vi "LDLT-Decomposition.vi"(11 "Input Matrix":T1) -> (2 "D":T1, 3 "L":T1)   [LabVIEW 2019]
doc: "This VI computes the square root free Cholesky factorization\n\n A=L*D*L'\n\nWhere L is a lower triangular matrix with ones on the diagonal, and D is a diagonal matrix. \nIt is assumed that A is symmetric and postive definite.\nReference: Golub and Van Loan, \"Matrix Computations\", second edition, p 137. \nit is based in the work made by Brian Borchers (borchers@nmt.edu) in MATLAB.\n\nCreated by Davis Montenegro\n10-05-2013"
uses:
  <vilib>/Analysis/Matrix/Datatypes/RealMatrix.ctl
  <vilib>/Analysis/Matrix/Numeric/Conversions/Matrix To Array - RM.vi
  <vilib>/Analysis/Matrix/Numeric/Conversions/Array To Matrix - RA.vi
  <vilib>/Analysis/Matrix/Numeric/Multiply/Multiply - RM,RM.vi
  <vilib>/Analysis/Matrix/Numeric/Subtract/Subtract (Elementwise) - R,RM.vi
  <vilib>/Analysis/Matrix/Numeric/Conversions/Array To Matrix - RA2.vi
  <vilib>/Analysis/Matrix/Numeric/Subtract/Subtract - RM,RM.vi
  <vilib>/Analysis/Matrix/NI_Matrix.lvlib
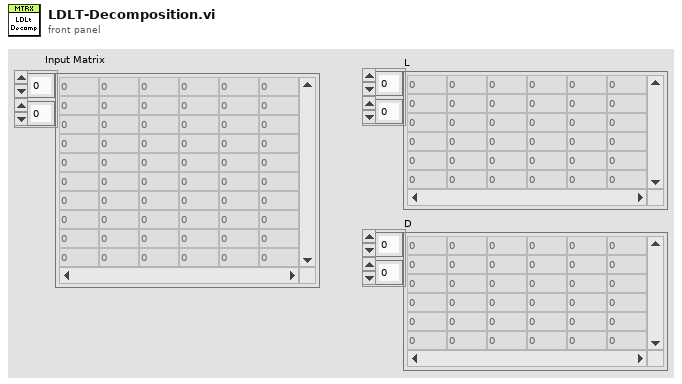
[diagram p1: front panel]
types:
  T1 = typedef "NI_Matrix.lvlib/RealMatrix.ctl" = dbl[][]
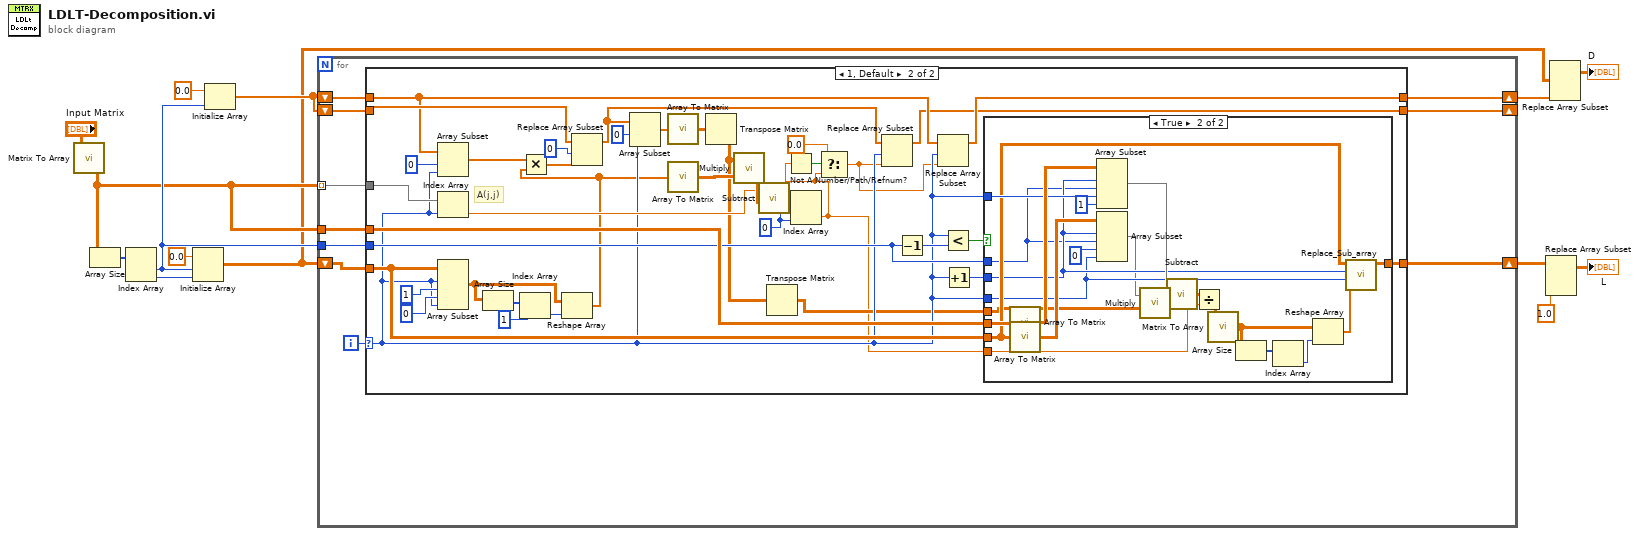
[diagram p0: block diagram]
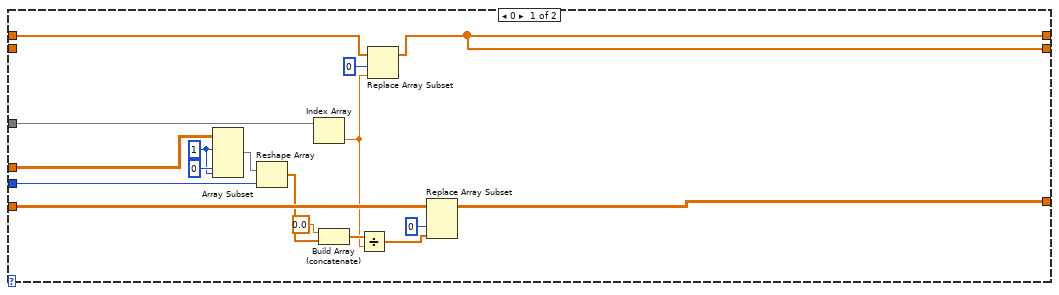
[diagram p2: hidden frame]
diagram:
  n1 = call-poly <vilib>:"Matrix To Array.vi"("Real Matrix"="Input Matrix") -> ("Real 2D Array"=w5:dbl[][])
  n2 = Array Size(array=w5) -> (size(s)=w14:i32[])
  n3 = Index Array(array=w14) -> (element #1=w10:i32, element #2=w13:i32)  [unwired: 2 in]
  n4 = Initialize Array(0.0, w10, w13) -> (w2:dbl[][])
  n5 = Initialize Array(0.0, w10) -> (w7:dbl[])
  n6 = for {
    tunnel: w5 -> [w23] mode=indexing
    shift-right: [w16] -> _
    shift-left: w7 -> [w22]
    shift-right: [w15] -> w3
    shift-left: w7 -> [w21]
    tunnel: w5 -> [w19]
    tunnel: w10 -> [w18]
    shift-right: [w17] -> w9
    shift-left: w2 -> [w20]
    i -> [w24]
    n7 = case shown="1, Default" w24 {
      selector: w24 -> [_ w52]
      tunnel: w23 -> [w41 w76]
      tunnel: w22 -> [_ w75]
      tunnel: w21 -> [w28 w68]
      tunnel: [w25 w67] -> w15
      tunnel: [w25 w50] -> w16
      tunnel: w20 -> [w37 w58]
      tunnel: w19 -> [w40 w65]
      tunnel: w18 -> [w33 w53]
      tunnel: [w31 w62] -> w17
      frame 0 {
        w38 = 1 ("index")
        n8 = Array Subset(array=w40, index (row)=w38, index (col)=0 ("index"), length (col)=w38) -> (w34:dbl[][])  [unwired: 1 in]
        n9 = Reshape Array(w34, w33) -> (w32:dbl[])
        n10 = Index Array(array=w41) -> (element=w26:dbl)  [unwired: 1 in]
        n11 = Build Array (concatenate)(0.0, w32) -> (w30:dbl[])
        n12 = Divide(x=w30, y=w26) -> (x/y=w29:dbl[])
        n13 = Replace Array Subset(array=w28, new element=w26, index=0 ("index (row)")) -> (w25:dbl[])
        n14 = Replace Array Subset(array=w37, new element=w29, index (col)=0 ("disabled index (col)")) -> (w31:dbl[][])  [unwired: 1 in]
      }
      frame 1, Default {
        w69 = 0 ("index (row)")
        # "A(j,j)"
        n15 = Array Subset(array=w68, index=0, length=w52) -> (w80:dbl[])
        n16 = Index Array(array=w76, index=w52) -> (element=w71:dbl)
        n17 = Array Subset(array=w58, index (row)=w52, length (row)=1 ("length"), index (col)=0 ("length"), length (col)=w52) -> (w77:dbl[][])
        n18 = Array Size(array=w77) -> (size(s)=w79:i32[])
        n19 = Index Array(array=w79, index=1) -> (element=w78:i32)
        n20 = Reshape Array(w77, w78) -> (w42:dbl[])
        n21 = Multiply(x=w80, y=w42) -> (x*y=w74:dbl[])
        n22 = Replace Array Subset(array=w75, new element=w74, index=0) -> (w56:dbl[])
        n23 = Array Subset(array=w56, index=0, length=w52) -> (w54:dbl[])
        n24 = call-poly <vilib>:"Array To Matrix.vi"("Real 1D Array"=w54) -> ("Real Matrix (Column Vector)"=w57:T1)
        n25 = call-poly <vilib>:"Array To Matrix.vi"("Real 1D Array"=w42) -> ("Real Matrix (Column Vector)"=w49:T1)
        n26 = Transpose Matrix(1:w57) -> (0:w48:T1)
        n27 = call-poly <vilib>:"Multiply.vi"("Real Matrix B"=w49, "Real Matrix A"=w48) -> ("A * B"=w72:T1)
        n28 = call-poly <vilib>:"Subtract.vi"("Real Matrix A"=w72, "Real Scalar c"=w71) -> ("c - A"=w70:T1)
        n29 = Transpose Matrix(1:w48) -> (0:w47:T1)
        n30 = Index Array(array=w70, index (row)=w69, index (col)=w69) -> (element=w44:dbl)
        n31 = Not A Number/Path/Refnum?(number/path/refnum=w44) -> (NaN/Path/Refnum?=w45:bool)
        n32 = Select(t=0.0, s=w45, f=w44) -> (s? t:f=w43:dbl)
        n33 = Replace Array Subset(array=w56, new element=w43, index=w52) -> (w50:dbl[])
        n34 = Decrement(x=w53) -> (x-1=w63:i32)
        n35 = Replace Array Subset(array=w68, new element=w43, index=w52) -> (w67:dbl[])
        n36 = Less?(x=w52, y=w63) -> (x < y?=w66:bool)
        n37 = Increment(x=w52) -> (x+1=w64:i32)
        n38 = case shown="True" w66 {
          tunnel: w58 -> [w81 w87]
          tunnel: w65 -> [_ w101]
          tunnel: w47 -> [_ w83]
          tunnel: w52 -> [_ w85]
          tunnel: w64 -> [_ w86]
          tunnel: w52 -> [_ w99]
          tunnel: w44 -> [_ w97]
          tunnel: [w81 w89] -> w62
          tunnel: w53 -> [_ w82]
          frame False {
          }
          frame True {
            n39 = call-poly <vilib>:"Array To Matrix.vi"("Real 2D Array"=w101) -> ("Real Matrix"=w100:T1)
            n40 = call-poly <vilib>:"Array To Matrix.vi"("Real 2D Array"=w87) -> ("Real Matrix"=w103:T1)
            n41 = Array Subset(array=w100, index (row)=w86, length (row)=w82, index (col)=w99, length (col)=1 ("length")) -> (w98:T1)
            n42 = Array Subset(array=w103, index (row)=w86, length (row)=w82, index (col)=0 ("index"), length (col)=w85) -> (w84:T1)
            n43 = call-poly <vilib>:"Multiply.vi"("Real Matrix B"=w83, "Real Matrix A"=w84) -> ("A * B"=w96:T1)
            n44 = call-poly <vilib>:"Subtract.vi"("Real Matrix B"=w96, "Real Matrix A"=w98) -> ("A - B"=w95:T1)
            n45 = Divide(x=w95, y=w97) -> (x/y=w93:T1)
            n46 = call-poly <vilib>:"Matrix To Array.vi"("Real Matrix"=w93) -> ("Real 2D Array"=w90:dbl[][])
            n47 = Array Size(array=w90) -> (size(s)=w92:i32[])
            n48 = Index Array(array=w92) -> (element=w91:i32)  [unwired: 1 in]
            n49 = Reshape Array(w90, w91) -> (w88:dbl[])
            n50 = call "Replace_Sub_array.vi"("Vector"=w88, "Index Column"=w85, "Index Row"=w86, "Array"=w87) -> ("New Array"=w89:dbl[][])  [unwired: 7 in]
          }
        }
      }
    }
  }
  n51 = Replace Array Subset(array=w9, new element=1.0 ("new diagonal/fill element")) -> (→"L":T1)  [unwired: 2 in]
  n52 = Replace Array Subset(array=w2, new element=w3) -> (→"D":T1)  [unwired: 2 in]
